vi "Get_BoardInformation.vi"(5 "Device Number":T1, 7 "Update":bool) -> (2 "Board Information":T4 {"Board"."Hardware Revision" items=["navX-MXP"=33, "navX-Micro"=40]; "Omnimount Config" items=["DEFAULT", "X_UP", "X_DOWN", "Y_UP", "Y_DOWN", "Z_UP", "Z_DOWN"]})   [LabVIEW 2019]
doc: "This navX VI will return the current Board Information.\nWho Am I\nHardware Revision\nFirmware Major and Minor\nCapability\nOmnimount Config"
uses:
  <vilib>/Rock Robotics/WPI/ThirdParty/Sensors/navX/_TypeDefs/Flags/Z900_navX_Flags_HardwareRevTypeDef.ctl
  <vilib>/Rock Robotics/WPI/ThirdParty/Sensors/navX/_TypeDefs/Flags/Z900_navX_Flags_OmnimountConfigTypeDef.ctl
  <vilib>/Rock Robotics/WPI/ThirdParty/Sensors/navX/_TypeDefs/FRIC_navX_DeviceNumbersTypeDef.ctl
  <vilib>/Rock Robotics/WPI/ThirdParty/Sensors/navX/_TypeDefs/Z900_navX_DeviceRegisters.ctl
  <vilib>/Rock Robotics/WPI/ThirdParty/Sensors/navX/_TypeDefs/Flags/Z900_navX_Flags_CapabilityTypeDef.ctl
  <vilib>/Rock Robotics/WPI/ThirdParty/Sensors/navX/_Util/Z900_navX_Util_LittleEndian_to_BigEndian.vi
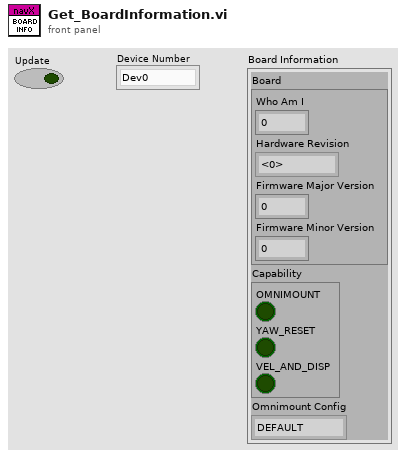
[diagram p1: front panel]
types:
  T1 = typedef "FRIC_navX_DeviceNumbersTypeDef.ctl" = enum16{"Dev0", "Dev1", "Dev2", "Dev3"}
  T2 = typedef "Z900_navX_Flags_HardwareRevTypeDef.ctl" = u8
  T3 = typedef "Z900_navX_Flags_OmnimountConfigTypeDef.ctl" = u8
  T4 = cluster{"Board":cluster{"Who Am I":u8, "Hardware Revision":T2, "Firmware Major Version":u8, "Firmware Minor Version":u8}, "Capability":cluster{"OMNIMOUNT":bool, "YAW_RESET":bool, "VEL_AND_DISP":bool}, "Omnimount Config":T3}
  T5 = cluster{"OMNIMOUNT":bool, "YAW_RESET":bool, "VEL_AND_DISP":bool}
  T6 = cluster{"Who Am I":u8, "Hardware Revision":T2, "Firmware Major Version":u8, "Firmware Minor Version":u8}
  T7 = typedef "Z900_navX_Flags_CapabilityTypeDef.ctl" = u16
  T8 = typedef "Z900_navX_DeviceRegisters.ctl" = u8
  T9 = cluster{"Board":cluster{"Who Am I":u8, "Hardware Revision":T2, "Firmware Major Version":u8, "Firmware Minor Version":u8}, "Capability":cluster{"OMNIMOUNT":bool, "YAW_RESET":bool, "VEL_AND_DISP":bool}, "Omnimount Config":T3}[]
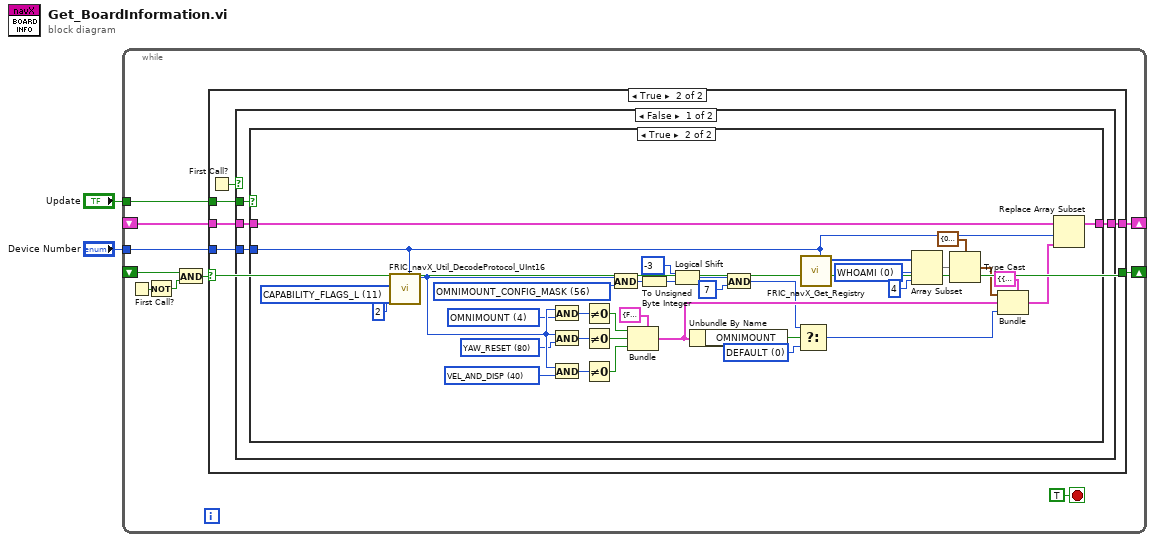
[diagram p0: block diagram]
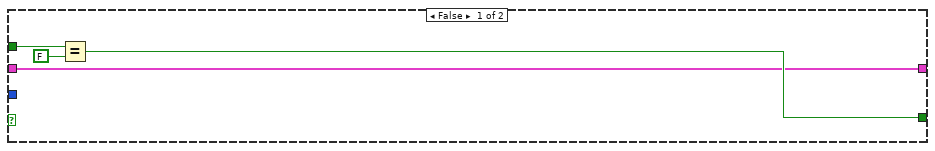
[diagram p2: hidden frame]
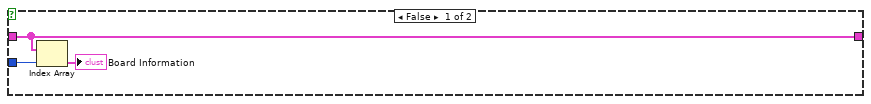
[diagram p3: hidden frame]
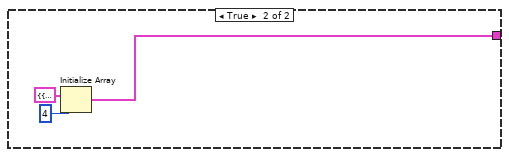
[diagram p4: hidden frame]
diagram:
  n1 = while {
    shift-right: [w12] -> _
    shift-left: _ -> [w11]
    tunnel: "Update" -> [w10]
    tunnel: "Device Number" -> [w8]
    shift-right: [w3] -> _
    shift-left: _ -> [w4]
    stop <- TRUE stop-if-true
    n2 = First Call?() -> (First Call?: T/F=w6:bool)
    n3 = Not(x=w6) -> (.not. x?=w7:bool)
    n4 = And(x=w4, y=w7) -> (x .and. y?=w5:bool)
    n5 = case shown="True" w5 {
      selector: w5 -> [_ w17]
      tunnel: [w13 w22] -> w12
      tunnel: w11 -> [w13 w21]
      tunnel: w10 -> [w15 w20]
      tunnel: w8 -> [_ w19]
      tunnel: [w14 w17] -> w3
      frame False {
        n6 = Equal?(x=w15, y=FALSE) -> (x = y?=w14:bool)
      }
      frame True {
        n7 = First Call?() -> (First Call?: T/F=w18:bool)
        n8 = case shown="False" w18 {
          tunnel: [w26 w65] -> w22
          tunnel: w21 -> [w25 _]
          tunnel: w20 -> [w24 _]
          tunnel: w19 -> [w23 _]
          frame False {
            n9 = case shown="True" w24 {
              tunnel: [w28 w52] -> w26
              tunnel: w25 -> [w28 w53]
              tunnel: w23 -> [w27 w50]
              frame False {
                n10 = Index Array(array=w28, index=w27) -> (element=→"Board Information":T4)
              }
              frame True {
                w38 = T7 56 items=["OMNIMOUNT"=4, "OMNIMOUNT_CONFIG_MASK"=56, "VEL_AND_DISP"=64, "YAW_RESET"=128] ("Capability Flag")
                w32 = u8 0 items=["DEFAULT", "X_UP", "X_DOWN", "Y_UP", "Y_DOWN", "Z_UP", "Z_DOWN"] ("OMNIMOUNT_CONFIG")
                w43 = T7 40 items=["OMNIMOUNT"=4, "OMNIMOUNT_CONFIG_MASK"=38, "VEL_AND_DISP"=40, "YAW_RESET"=80] ("Capability Flag")
                w44 = T7 80 items=["OMNIMOUNT"=4, "OMNIMOUNT_CONFIG_MASK"=38, "VEL_AND_DISP"=40, "YAW_RESET"=80] ("Capability Flag")
                w49 = T7 4 items=["OMNIMOUNT"=4, "OMNIMOUNT_CONFIG_MASK"=38, "VEL_AND_DISP"=40, "YAW_RESET"=80] ("Capability Flag")
                w54 = T8 0 items=["WHOAMI"=0, "HW_REV"=1, "FW_VER_MAJOR"=2, "FW_VER_MINOR"=3, "UPDATE_RATE_HZ"=4, "ACCEL_FSR_G"=5, "GYRO_FSR_DPS"=6, "OP_STATUS"=8, "CAL_STATUS"=9, "SELFTEST_STATUS"=10, "CAPABILITY_FLAGS_L"=11, "CAPABILITY_FLAGS_H"=12, "SENSOR_STATUS"=16, "TIMESTAMP"=18, "YAW"=22, "ROLL"=24, "PITCH"=26, "HEADING"=28, "FUSED_HEADING"=30, "ALTITUDE_I"=32, "ALTITUDE_D"=34, "LINERA_ACC_X"=36, "LINERA_ACC_Y"=38, "LINERA_ACC_Z"=40, "QUAT_W"=42, "QUAT_X"=44, "QUAT_Y"=46, "QUAT_Z"=48, "MPU_TEMP_C"=50, "GYRO_X"=52, "GYRO_Y"=54, "GYRO_Z"=56, "ACC_X"=58, "ACC_Y"=60, "ACC_Z"=62, "MAG_X"=64, "MAG_Y"=66, "MAG_Z"=68, "PRESSURE_I"=70, "PRESSURE_D"=72, "PRESSURE_TEMP"=74, "YAW_OFFSET"=76, "QUAT_OFFSET_W"=78, "QUAT_OFFSET_X"=80, "QUAT_OFFSET_Y"=82, "QUAT_OFFSET_Z"=84, "INTEGRATION_CONTROL"=86, "VELOCITY_X"=88, "VELOCITY_Y"=92, "VELOCITY_Z"=96, "DISPLACMENT_X"=100, "DISPLACMENT_Y"=104, "DISPLACEMENT_Z"=108] ("Device Register")
                w58 = T8 11 items=["WHOAMI"=0, "HW_REV"=1, "FW_VER_MAJOR"=2, "FW_VER_MINOR"=3, "UPDATE_RATE_HZ"=4, "ACCEL_FSR_G"=5, "GYRO_FSR_DPS"=6, "OP_STATUS"=8, "CAL_STATUS"=9, "SELFTEST_STATUS"=10, "CAPABILITY_FLAGS_L"=11, "CAPABILITY_FLAGS_H"=12, "SENSOR_STATUS"=16, "TIMESTAMP"=18, "YAW"=22, "ROLL"=24, "PITCH"=26, "HEADING"=28, "FUSED_HEADING"=30, "ALTITUDE_I"=32, "ALTITUDE_D"=34, "LINERA_ACC_X"=36, "LINERA_ACC_Y"=38, "LINERA_ACC_Z"=40, "QUAT_W"=42, "QUAT_X"=44, "QUAT_Y"=46, "QUAT_Z"=48, "MPU_TEMP_C"=50, "GYRO_X"=52, "GYRO_Y"=54, "GYRO_Z"=56, "ACC_X"=58, "ACC_Y"=60, "ACC_Z"=62, "MAG_X"=64, "MAG_Y"=66, "MAG_Z"=68, "PRESSURE_I"=70, "PRESSURE_D"=72, "PRESSURE_TEMP"=74, "YAW_OFFSET"=76, "QUAT_OFFSET_W"=78, "QUAT_OFFSET_X"=80, "QUAT_OFFSET_Y"=82, "QUAT_OFFSET_Z"=84, "INTEGRATION_CONTROL"=86, "VELOCITY_X"=88, "VELOCITY_Y"=92, "VELOCITY_Z"=96, "DISPLACMENT_X"=100, "DISPLACMENT_Y"=104, "DISPLACEMENT_Z"=108] ("Device Register")
                n11 = call <vilib>:"FRIC_navX_Util_DecodeProtocol_UInt16.vi"("Device Number"=w50, "length"=2, "Device Register"=w58) -> ("Value"=w56:u16)  [unwired: 8 in]
                n12 = And(x=w56, y=w49) -> (x .and. y?=w48:T7)
                n13 = And(x=w56, y=w44) -> (x .and. y?=w45:T7)
                n14 = And(x=w56, y=w43) -> (x .and. y?=w42:T7)
                n15 = Not Equal To 0?(x=w48) -> (x != 0?=w46:bool)
                n16 = Not Equal To 0?(x=w45) -> (x != 0?=w41:bool)
                n17 = Not Equal To 0?(x=w42) -> (x != 0?=w40:bool)
                n18 = And(x=w56, y=w38) -> (x .and. y?=w37:T7)
                n19 = Bundle(cluster=T5 {"OMNIMOUNT"=FALSE, "YAW_RESET"=FALSE, "VEL_AND_DISP"=FALSE}, "OMNIMOUNT"=w46, "YAW_RESET"=w41, "VEL_AND_DISP"=w40) -> (w60:T5)
                n20 = To Unsigned Byte Integer(number=w37) -> (unsigned 8bit integer=w33:u8)
                n21 = Logical Shift(y=-3, x=w33) -> (x << y=w35:u8)
                n22 = Unbundle By Name(w60) -> ("OMNIMOUNT"=w39:bool)
                n23 = And(x=w35, y=7) -> (x .and. y?=w31:i32)
                n24 = Select(t=w31, s=w39, f=w32) -> (s? t:f=w30:i32)
                n25 = call <vilib>:"FRIC_navX_Get_Registry.vi"("Device Number"=w50) -> ("Registry (out)"=w64:u8[])  [unwired: 9 in, 1 out]
                n26 = Array Subset(array=w64, index=w54, length=4) -> (w63:u8[])
                n27 = Type Cast(type=T6 {"Who Am I"=0, "Hardware Revision"=33, "Firmware Major Version"=0, "Firmware Minor Version"=0}, x=w63) -> (*(type *) &x=w59:T6)
                n28 = Bundle(cluster=T4 {"Board"={"Who Am I"=0, "Hardware Revision"=33, "Firmware Major Version"=0, "Firmware Minor Version"=0}, "Capability"={"OMNIMOUNT"=FALSE, "YAW_RESET"=FALSE, "VEL_AND_DISP"=FALSE}, "Omnimount Config"=0}, "Board"=w59, "Capability"=w60, "Omnimount Config"=w30) -> (w51:T4)
                n29 = Replace Array Subset(array=w53, new element=w51, index=w50) -> (w52:T9)
              }
            }
          }
          frame True {
            n30 = Initialize Array(T4 {"Board"={"Who Am I"=0, "Hardware Revision"=0, "Firmware Major Version"=0, "Firmware Minor Version"=0}, "Capability"={"OMNIMOUNT"=FALSE, "YAW_RESET"=FALSE, "VEL_AND_DISP"=FALSE}, "Omnimount Config"=0}, 4 ("dimension size")) -> (w65:T9)
          }
        }
      }
    }
  }
